vi "Find Entity by Type.vi"(7 "Entity Type":refnum<class "Entity.lvclass">, 8 "error in (no error)":errorcluster, 10 "Type":refnum<class "Type.lvclass">, 11 "Entity Manager in":refnum<class "Entity Manager.lvclass">) -> (0 "error out":errorcluster, 2 "Entity":refnum<class "Entity.lvclass">, 3 "Entity Manager out":refnum<class "Entity Manager.lvclass">)   [LabVIEW 2020, in "Conditum.lvlib" / "Entity Manager.lvclass"]
uses:
  Entity Manager.lvclass
  Entity Manager.lvclass/Entity Manager.ctl
  Database Platform/Database Platform.lvclass
  Unit Of Work Session/Unit Of Work Session.lvclass
  Entity/Entity.lvclass
  Columns/Type/Type.lvclass
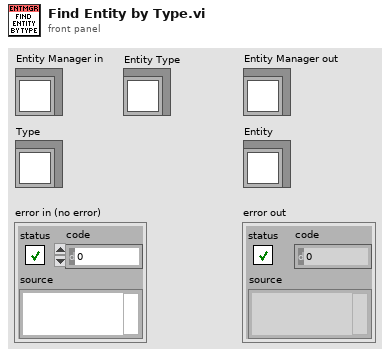
[diagram p1: front panel]
types:
  T1 = typedef "Conditum.lvlib/Entity Manager.lvclass/Known Entity.ctl" = cluster{"Entity":refnum<class "Entity.lvclass">, "Types":refnum<class "Type.lvclass">[], "Type Name Map":map{string, i32}}
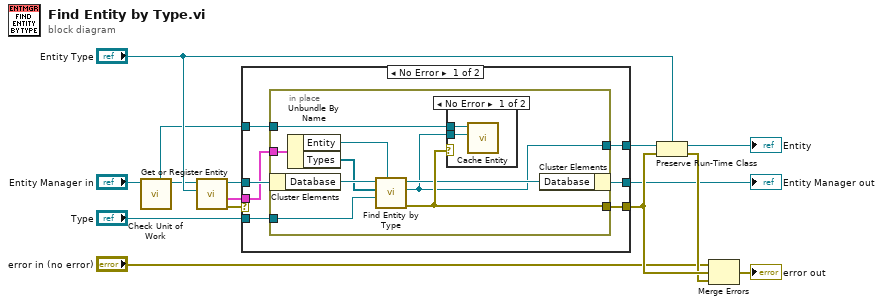
[diagram p0: block diagram]
diagram:
  n1 = call "Check Unit of Work.vi"("Entity Manager in"="Entity Manager in") -> ("Entity Manager out"=w2:refnum<class "Entity Manager.lvclass">, "Unit Of Work"=w1:refnum<class "Unit Of Work Session.lvclass">)  [unwired: 8 in, 1 out]
  n2 = call "Get or Register Entity.vi"("Entity"="Entity Type", "Entity Manager in"=w2) -> ("error out"=w6:errorcluster, "Entity Info"=w10:T1, "Entity Manager out"=w11:refnum<class "Entity Manager.lvclass">)  [unwired: 7 in]
  n3 = case shown="No Error" w6 {
    selector: w6 -> [_ w35]
    tunnel: [w22 w35] -> w15
    tunnel: "Type" -> [w21 _]
    tunnel: [w20 w34] -> w12
    tunnel: w11 -> [w19 w34]
    tunnel: w10 -> [w18 _]
    tunnel: [w17 _] -> w9
    tunnel: w1 -> [w16 _]
    frame No Error {
      n4 = in-place {
        in-place-border: w21 -> [w28]
        in-place-border: [w31] -> w22
        in-place-border: w18 -> [w27]
        in-place-border: [w23] -> w17
        in-place-border: w16 -> [w24]
        n5 = in-place-cluster #1(w19) -> ("Database"=w30:refnum<class "Database Platform.lvclass">)
        n6 = Unbundle By Name(w27) -> ("Entity"=w26:refnum<class "Entity.lvclass">, "Types"=w25:refnum<class "Type.lvclass">[])
        n7 = call "Find Entity by Type.vi"("Entity Type"=w26, "Column Criteria"=w28, "Types"=w25, "Database in"=w30) -> ("error out"=w31:errorcluster, "Entity"=w23:refnum<class "Entity.lvclass">, "Database out"=w29:refnum<class "Database Platform.lvclass">)  [unwired: 5 in]
        n8 = case shown="No Error" w31 {
          tunnel: w24 -> [w33 _]
          tunnel: w23 -> [w32 _]
          frame No Error {
            n9 = call "Cache Entity.vi"("Conditum:Entity"=w32, "Unit Of Work in"=w33) -> ()  [unwired: 9 in, 1 out]
          }
          frame Error {
          }
        }
        n10 = in-place-cluster #1("Database"=w29) -> (w20:refnum<class "Entity Manager.lvclass">)
      }
    }
    frame Error {
    }
  }
  "Entity Manager out" <- w12
  n11 = Preserve Run-Time Class(object in=w9, error in=w15, 2:"Entity Type") -> (object out=→"Entity":refnum<class "Entity.lvclass">, error out=w14:errorcluster)
  n12 = Merge Errors("error in (no error)", w15, w14) -> (→"error out":errorcluster)
